vi "Main.vi"(4 "Start":bool, 6 "Name":string, 8 "Time Stamp":timestamp format="%<%x>T", 10 "Next":bool, 11 "Error in":errorcluster) -> (15 "Error out":errorcluster)   [LabVIEW 2020]
doc: "This is a game which is used to test for personality of a person"
panel:
  out "Status":string
  in  "Password":string
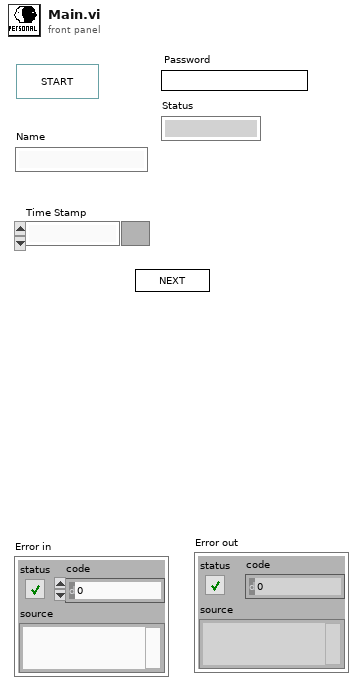
[diagram p1: front panel]
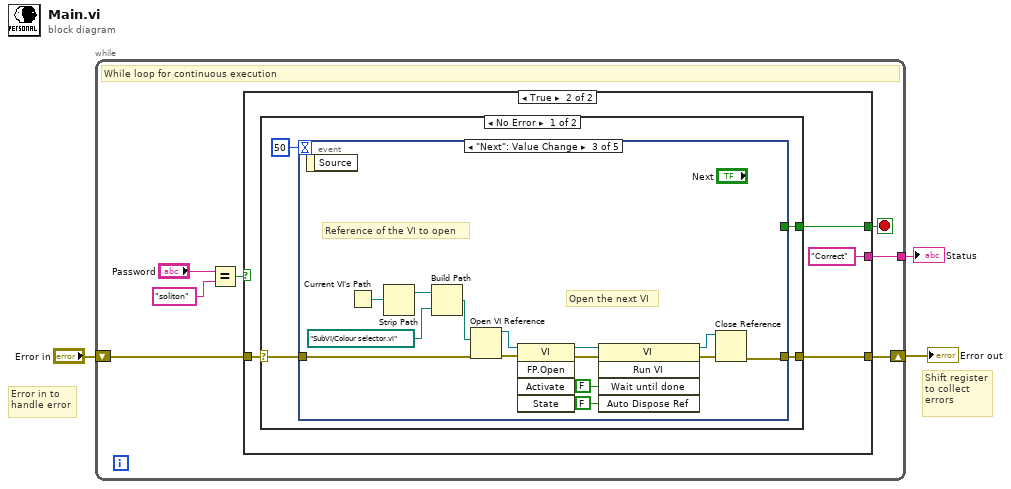
[diagram p0: block diagram]
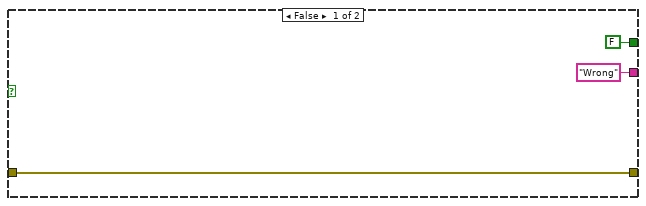
[diagram p2: hidden frame]
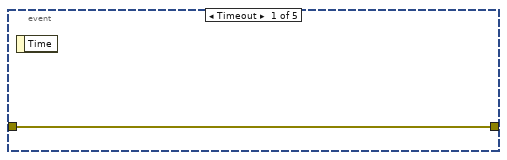
[diagram p3: hidden frame]
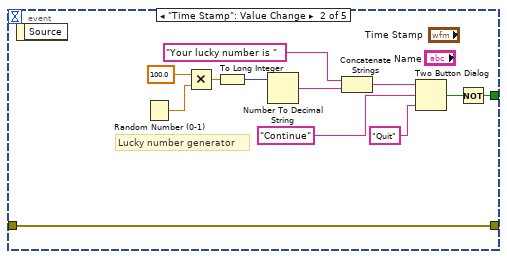
[diagram p4: hidden frame]
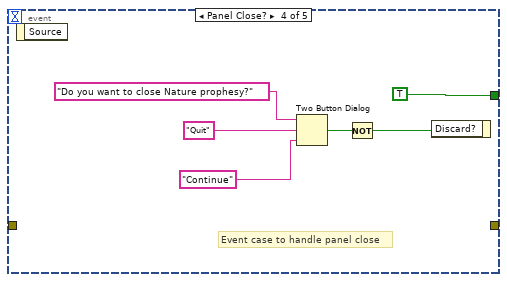
[diagram p5: hidden frame]
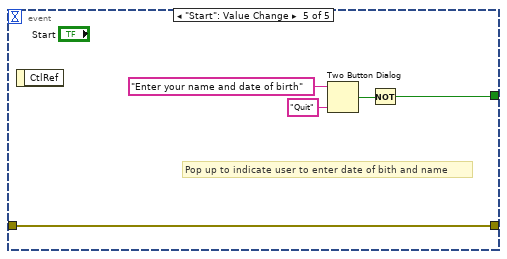
[diagram p6: hidden frame]
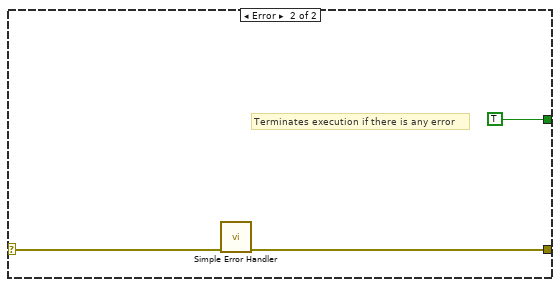
[diagram p7: hidden frame]
diagram:
  # "Shift register\nto collect \nerrors"
  # "Error in to\nhandle error"
  n1 = while {
    shift-right: [w9] -> w2
    shift-left: "Error in" -> [w10]
    tunnel: [w4] -> w1
    stop <- w8 stop-if-true
    # "While loop for continuous execution"
    n2 = Equal?(x="Password", y="soliton") -> (x = y?=w5:bool)
    n3 = case shown="True" w5 {
      tunnel: w10 -> [w11 w17]
      tunnel: [w11 w16] -> w9
      tunnel: [FALSE w15] -> w8
      tunnel: ["Wrong" ("Status") "Correct" ("Status")] -> w4
      frame False {
      }
      frame True {
        n4 = case shown="No Error" w17 {
          selector: w17 -> [w21 w62]
          tunnel: [w20 w61] -> w16
          tunnel: [w18 TRUE] -> w15
          frame No Error {
            n5 = event shown="[2] \"Next\": Value Change" {
              selector: _ -> [_ _ _ _ _]
              dyn-events: _ -> [_ _ _ _ _]
              timeout: 50 -> [_ _ _ _ _]
              tunnel: w21 -> [w22 w23 w41 _ w59]
              tunnel: [w22 w23 w35 _ w59] -> w20
              tunnel: [_ w24 _ TRUE w55] -> w18
              event Timeout {
                n6 = event-data() -> ()  [unwired: 1 in, 1 out]
              }
              event "Time Stamp": Value Change {
                # "Lucky number generator"
                n7 = event-data() -> ()  [unwired: 1 in, 1 out]
                n8 = Random Number (0-1)() -> (number: 0 to 1=w33:dbl)
                n9 = Multiply(x=100.0, y=w33) -> (x*y=w32:dbl)
                n10 = To Long Integer(number=w32) -> (32bit integer=w31:i32)
                n11 = Number To Decimal String(number=w31) -> (decimal integer string=w30:string)  [unwired: 1 in]
                n12 = Concatenate Strings("Your lucky number is ", w30) -> (w28:string)
                n13 = Two Button Dialog(message=w28, 1:"Quit" ("F button name (\"Cancel\")"), 2:"Continue" ("T button name (\"OK\")")) -> (T button?=w26:bool)
                n14 = Not(x=w26) -> (.not. x?=w24:bool)
              }
              event "Next": Value Change {
                # "Open the next VI"
                # "Reference of the VI to open"
                n15 = event-data() -> ()  [unwired: 1 in, 1 out]
                n16 = Current VI's Path() -> (path=w47:path)
                n17 = Strip Path(path=w47) -> (stripped path=w40:path)  [unwired: 1 out]
                n18 = Build Path(base path=w40, name or relative path=path "SubVI/Colour selector.vi") -> (appended path=w46:path)
                n19 = Open VI Reference(vi path=w46, error in (no error)=w41) -> (vi reference=w45:refnum<vi>, error out=w44:errorcluster)  [unwired: 4 in]
                n20 = invoke class="VI" method="FP.Open"(reference=w45, error in=w44) -> (reference out=w43:refnum<vi>, error out=w42:errorcluster)  [unwired: 3 in, 3 out]
                n21 = invoke class="VI" method="Run VI"(reference=w43, error in=w42, "Wait until done"=FALSE ("Wait Until Done"), "Auto Dispose Ref"=FALSE ("Auto Dispose Reference")) -> (reference out=w37:refnum<vi>, error out=w36:errorcluster)  [unwired: 1 in, 3 out]
                n22 = Close Reference(reference=w37, error in (no error)=w36) -> (error out=w35:errorcluster)
              }
              event Panel Close? {
                # "Event case to handle panel close"
                n23 = event-data() -> ()  [unwired: 1 in, 1 out]
                n24 = Two Button Dialog(message="Do you want to close Nature prophesy?", 1:"Continue" ("F button name (\"Cancel\")"), 2:"Quit" ("T button name (\"OK\")")) -> (T button?=w53:bool)
                n25 = Not(x=w53) -> (.not. x?=w52:bool)
                n26 = event-data("Discard?"=w52) -> ()  [unwired: 1 in, 1 out]
              }
              event "Start": Value Change {
                # "Pop up to indicate user to enter date of bith and name"
                n27 = event-data() -> ()  [unwired: 1 in, 1 out]
                n28 = Two Button Dialog(message="Enter your name and date of birth", 1:"Quit" ("F button name (\"Cancel\")")) -> (T button?=w58:bool)  [unwired: 1 in]
                n29 = Not(x=w58) -> (.not. x?=w55:bool)
              }
            }
          }
          frame Error {
            # "Terminates execution if there is any error"
            n30 = call <vilib>:"Simple Error Handler.vi"("error in (no error)"=w62) -> ("error out"=w61:errorcluster)  [unwired: 4 in, 4 out]
          }
        }
      }
    }
  }
  "Status" <- w1
  "Error out" <- w2
